vi "Read I32.vi"(8 "error in (no error)":errorcluster, 9 "Default If Not Found":i32, 10 "Name":string, 11 "IConfiguration in":refnum<class "IConfiguration.lvclass">) -> (0 "error out":errorcluster, 1 "Not Found?":bool, 2 "Value":i32, 3 "IConfiguration out":refnum<class "IConfiguration.lvclass">)   [LabVIEW 2020, in "Configuration.lvlib" / "IConfiguration.lvclass"]
uses:
  <vilib>/gpm_packages/@cs/Configuration/Source/IConfiguration/IConfiguration.lvclass
  <vilib>/Utility/Data Type/Type Definitions/Data Type.ctl
  ece91c06-bf80-45f7-8a24-240eaa39dbde.vi
  <vilib>/Utility/error.llb/Error Cluster From Error Code.vi
  <vilib>/Utility/Data Type/NI_Data Type.lvlib
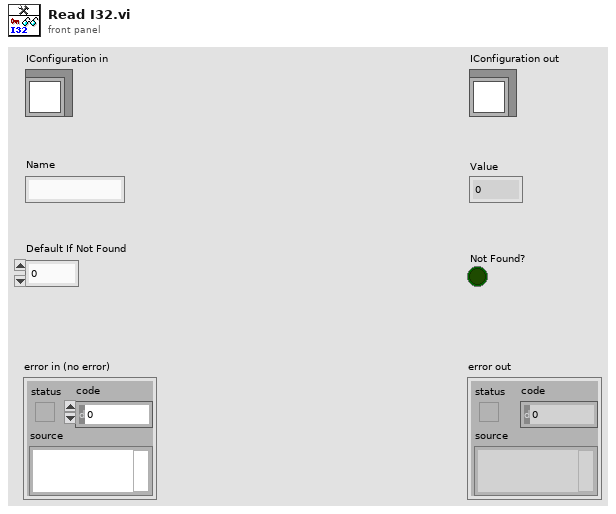
[diagram p1: front panel]
types:
  T1 = typedef "NI_Data Type.lvlib/Data Type.ctl" = enum8{"Invalid Type", "Void", "I8", "I16", "I32", "I64", "U8", "U16", "U32", "U64", "Single Float", "Double Float", "Extended Float", "Single Complex", "Double Complex", "Extended Complex", "Enum U8", "Enum U16", "Enum U32", "Enum U64", "Single Float With Unit", "Double Float With Unit", "Extended Float With Unit", "Single Complex with Unit", "Double Complex with Unit", "Extended Complex with Unit", "Boolean", "String", "Path", "Picture", "Tag", "Array", "Cluster", "Variant", "LV Variant", "Waveform", "Timestamp", "Digital Waveform", "Digital Data", "ExpressData", "Refnum", "External Data", "VI", "Poly VI", "LabVIEW Class Instance", "Fixed Point", "Set Collection", "Map Collection"}
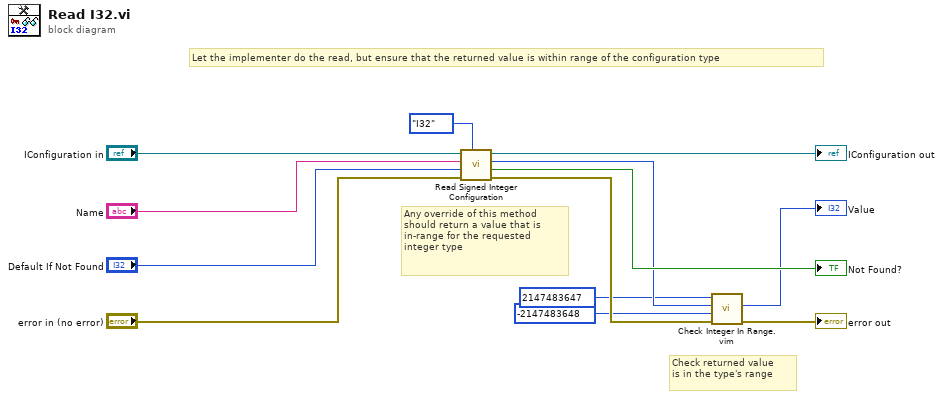
[diagram p0: block diagram]
diagram:
  # "Any override of this method\nshould return a value that is\nin-range for the requested\ninteger type"
  # "Check returned value\nis in the type's range"
  # "Let the implementer do the read, but ensure that the returned value is within range of the configuration type"
  n1 = call-dynamic "Read Signed Integer Configuration.vi"("Type"=Data_Type."I32", "error in (no error)"="error in (no error)", "Default If Not Found"="Default If Not Found", "Name"="Name", "IConfiguration in"="IConfiguration in") -> ("error out"=w6:errorcluster, "Not Found?"=→"Not Found?":bool, "Value"=w4:i64, "IConfiguration out"=→"IConfiguration out":refnum<class "IConfiguration.lvclass">)  [unwired: 3 in]
  n2 = call "Check Integer In Range.vim"("error in (no error)"=w6, "Lower Limit"=i64 -2147483648, "Value"=w4, "Upper Limit"=i64 2147483647) -> ("error out"=→"error out":errorcluster, "Coerced Value"=→"Value":i64)  [unwired: 6 in]
